vi "写入多个寄存器 (子VI).vi"(8 "错误输入（无错误）":errorcluster, 9 "holding register value":u16 caption="保持寄存器值", 10 "address":u16 caption="地址", 11 "VISA resource name":refnum<visa-resource-name> caption="VISA资源名称") -> (0 "错误输出":errorcluster)   [LabVIEW 2016, in "斯坦道CODMn.lvlib"]
uses:
  <vilib>/Modbus/master/Create Master Instance (Serial).vi
  <vilib>/Modbus/master/Modbus Master.lvclass
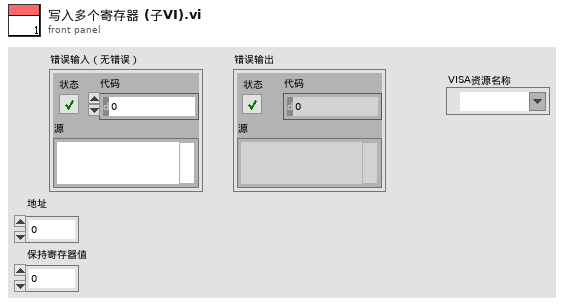
[diagram p1: front panel]
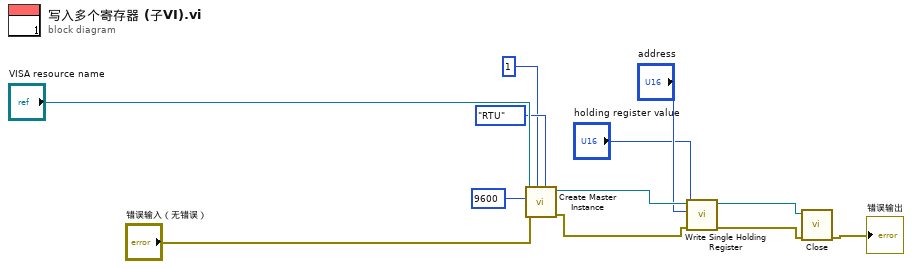
[diagram p0: block diagram]
diagram:
  n1 = call-poly <vilib>:"Create Master Instance.vi"("serial type"=enum16{"RTU", "ASCII"}."RTU", "unit ID"=u8 1, "error in (no error)"="错误输入（无错误）", "baud rate (9600)"=u32 9600, "VISA resource name"="VISA resource name") -> ("error out"=w7:errorcluster, "serial master instance"=w8:refnum<class "Modbus Master.lvclass">)  [unwired: 5 in]
  n2 = call-dynamic "Write Single Holding Register.vi"("error in (no error)"=w7, "holding register value"="holding register value", "address"="address", "Modbus master in"=w8) -> ("error out"=w5:errorcluster, "Modbus master out"=w6:refnum<class "Modbus Master.lvclass">)  [unwired: 6 in]
  n3 = call-dynamic "Close.vi"("error in (no error)"=w5, "Modbus master in"=w6) -> ("error out"=→"错误输出":errorcluster)  [unwired: 9 in]
